vi "PPMS.Open.vi"(8 "error in (no error)":errorcluster, 11 "instrument.PPMS in":refnum<class "instrument.PPMS.lvclass">) -> (0 "error out":errorcluster, 3 "instrument.PPMS out":refnum<class "instrument.PPMS.lvclass">)   [LabVIEW 2019, in "instrument.PPMS.lvclass"]
uses:
  instrument.PPMS.lvclass
  C:/Program Files (x86)/National Instruments/LabVIEW 2019/user.lib/LevyLab/Instrument Framework/Instrument/Instrument.lvclass
  <userlib>/LevyLab/Instrument Framework/Instrument/Instrument.lvclass/Instrument.ctl
  instrument.PPMS.lvclass/instrument.PPMS.ctl
  <userlib>/LevyLab/Instrument Framework/Instrument/Instrument.lvclass
  C:/Program Files (x86)/National Instruments/LabVIEW 2019/user.lib/LevyLab/Instrument Framework/Instrument Types/Cryostat/Instrument.Cryostat.lvclass
  C:/Program Files (x86)/National Instruments/LabVIEW 2019/vi.lib/JKI/JKI SMO/SMO/SMO.lvclass
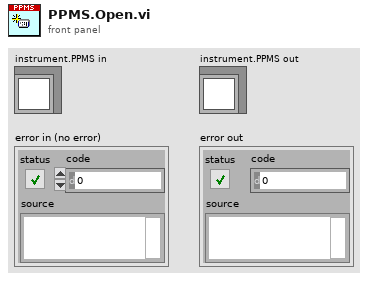
[diagram p1: front panel]
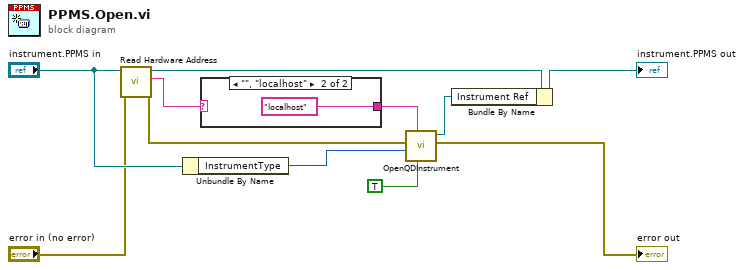
[diagram p0: block diagram]
diagram:
  n1 = call <userlib>:"Read Hardware Address.vi"("error in (no error)"="error in (no error)", "Instrument in"="instrument.PPMS in") -> ("error out"=w5:errorcluster, "Address"=w9:string, "Instrument out"=w4:refnum<class "instrument.PPMS.lvclass">)  [unwired: 7 in]
  n2 = Unbundle By Name("instrument.PPMS in") -> ("InstrumentType"=w1:i32)
  n3 = case shown="\"\", \"localhost\"" w9 {
    selector: w9 -> [w12 _]
    tunnel: [w12 "localhost" ("y")] -> w8
    frame Default {
    }
    frame "", "localhost" {
    }
  }
  n4 = call "OpenQDInstrument.vi"("Remote"=TRUE, "IP Address"=w8, "InstrumentType"=w1, "error in (no error)"=w5) -> ("error out"=→"error out":errorcluster, "Instrument Ref"=w7:refnum<k24>)  [unwired: 4 in]
  n5 = Bundle By Name(cluster=w4, "Instrument Ref"=w7) -> (→"instrument.PPMS out":refnum<class "instrument.PPMS.lvclass">)
